vi "Set Task.vi"(10 "Task":refnum<k21>, 11 "DAQmx Base CFG in":refnum<class "DAQmx Base CFG.lvclass">) -> (3 "DAQmx Base CFG out":refnum<class "DAQmx Base CFG.lvclass">)   [LabVIEW 2024, in "DAQmx Base CFG.lvclass"]
uses:
  DAQmx Base CFG.lvclass
  DAQmx Base CFG.lvclass/DAQmx Base CFG.ctl
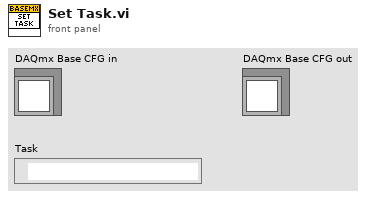
[diagram p1: front panel]
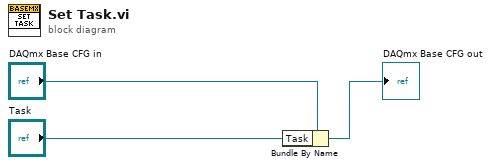
[diagram p0: block diagram]
diagram:
  n1 = Bundle By Name(cluster="DAQmx Base CFG in", "Task"="Task") -> (→"DAQmx Base CFG out":refnum<class "DAQmx Base CFG.lvclass">)
